vi "Load Notifier.vi"(0 "LVx.lvlib:LVx.lvclass":refnum<class "LVx.lvclass">, 7 "GUI Response Notifier":T1, 11 "error in (no error)":errorcluster) -> (4 "LVx.lvclass out":refnum<class "LVx.lvclass">, 8 "GUI Response Notifier":T1, 15 "error out":errorcluster)   [LabVIEW 2011, in "LVx.lvlib" / "LVx.lvclass"]
uses:
  LVx.lvclass
  TypeDef/Typedef - LVx Response Notifier.ctl
  LVx.lvclass/LVx.ctl
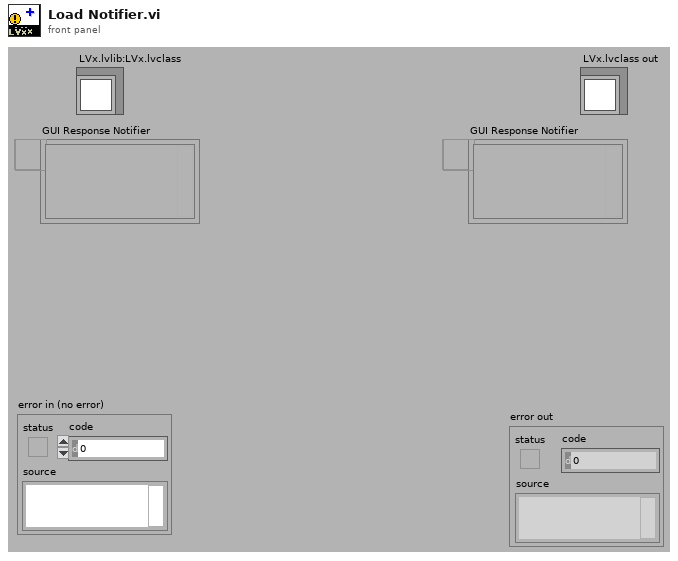
[diagram p1: front panel]
types:
  T1 = typedef "LVx.lvlib/LVx.lvclass/Typedef - LVx Response Notifier.ctl" = refnum<notifier>
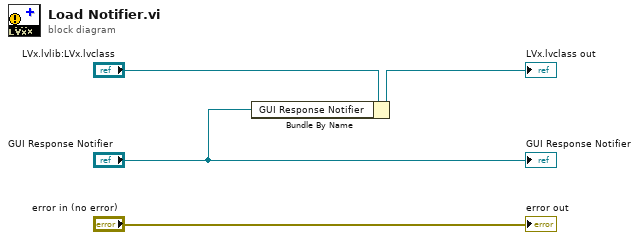
[diagram p0: block diagram]
diagram:
  n1 = Bundle By Name(cluster="LVx.lvlib:LVx.lvclass", "GUI Response Notifier"="GUI Response Notifier") -> (→"LVx.lvclass out":refnum<class "LVx.lvclass">)
  "error out" <- "error in (no error)"
  "GUI Response Notifier" <- "GUI Response Notifier"
